vi "Read URI.vi"(11 "ConfigManager in":refnum<class "ConfigManager.lvclass">) -> (2 "URI":string, 3 "ConfigManager out":refnum<class "ConfigManager.lvclass">)   [LabVIEW 2013, in "CfgManager.lvlib" / "ConfigManager.lvclass"]
uses:
  ConfigManager.lvclass
  ConfigManager.lvclass/ConfigManager.ctl
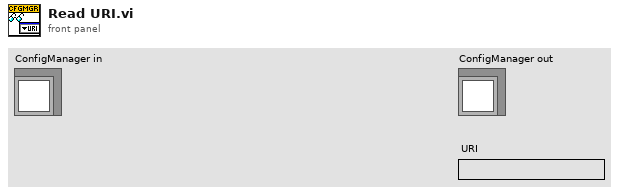
[diagram p1: front panel]
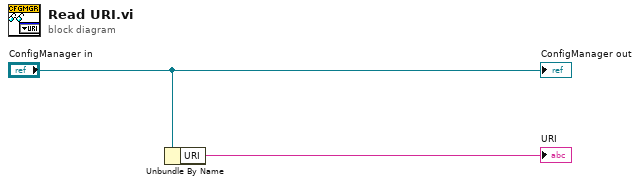
[diagram p0: block diagram]
diagram:
  n1 = Unbundle By Name("ConfigManager in") -> ("URI"=→"URI":string)
  "ConfigManager out" <- "ConfigManager in"
